vi "Save Direct Summing.vi"(6 "Direct Sum":dbl[](array[numeric]), 7 "Experimental parameters":dbl[](array[numeric]), 8 "Current File Num":u16, 9 "Best Fit Parameters":dbl[](array[numeric]), 10 "Fitting Results Save Path":string, 11 "Fitting Type":u16(ring)) -> ()   [LabVIEW 2015]
uses:
  <vilib>/Utility/file.llb/Read From Spreadsheet File (DBL).vi
  <vilib>/Utility/file.llb/Write To Spreadsheet File (DBL).vi
panel:
  out "Best Fit Parameters 2":dbl[](array[numeric])
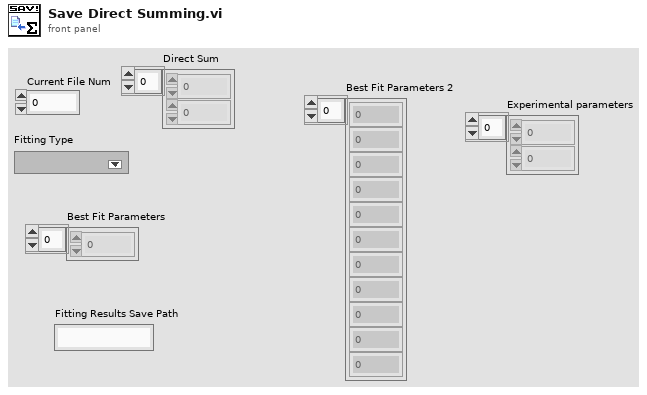
[diagram p1: front panel]
types:
  T1 = enum16{"open", "replace", "create", "open or create", "replace or create", "replace or create with confirmation"}
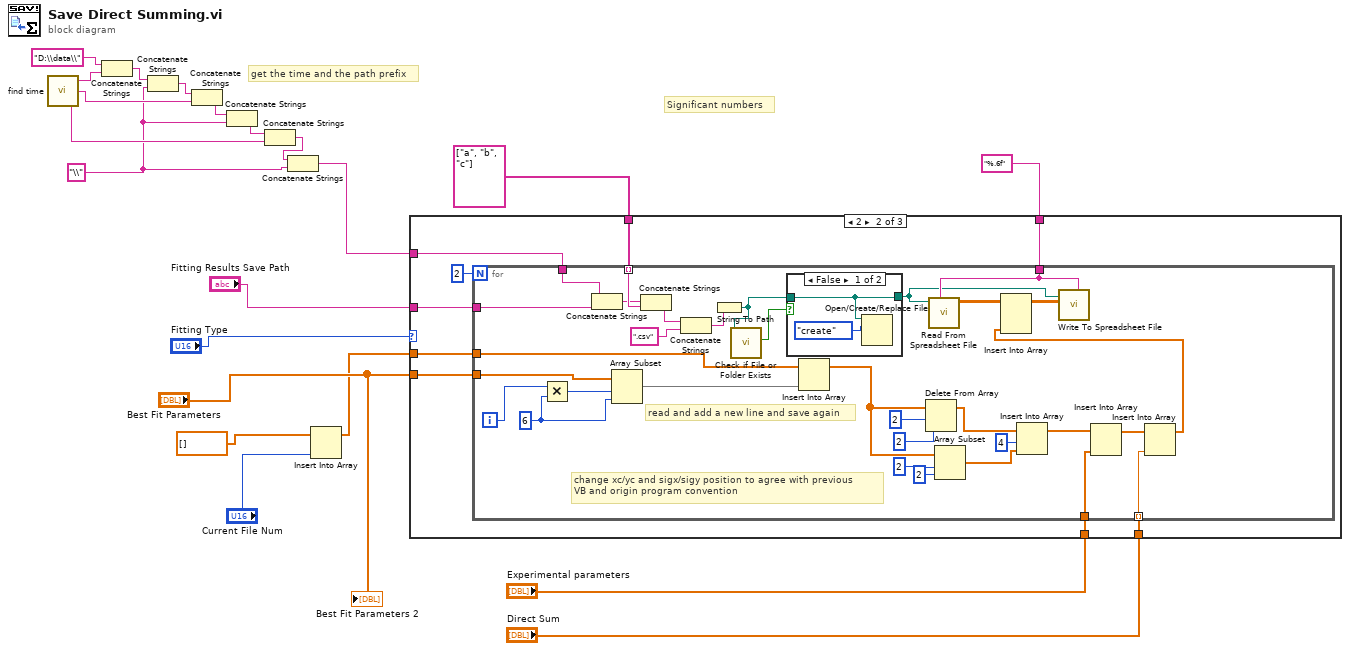
[diagram p0: block diagram]
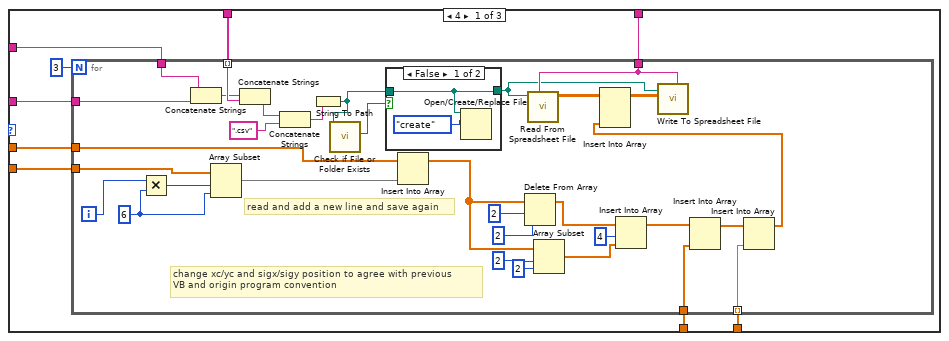
[diagram p2: hidden frame]
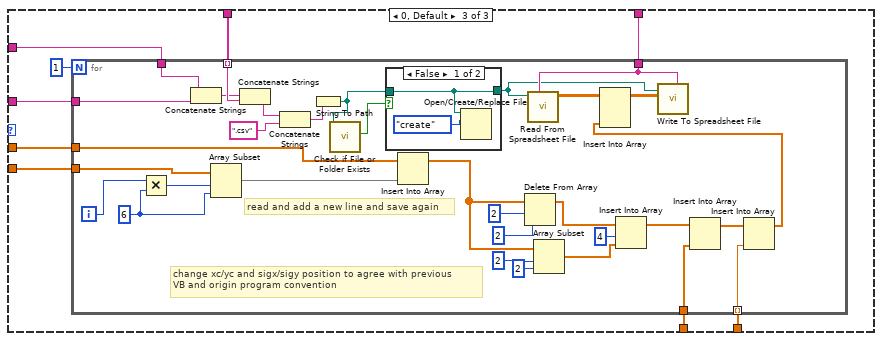
[diagram p5: hidden frame]
diagram:
  w5 = "\\" ("字符串")
  # "get the time and the path prefix"
  # "Significant numbers"
  n1 = call "find time.vi"() -> ("day"=w7:string, "month"=w10:string, "year"=w13:string)  [unwired: 3 in]
  n2 = Concatenate Strings("D:\\data\\", w13) -> (w12:string)
  n3 = Concatenate Strings(w12, w5) -> (w11:string)
  n4 = Concatenate Strings(w11, w10) -> (w9:string)
  n5 = Concatenate Strings(w9, w5) -> (w8:string)
  n6 = Concatenate Strings(w8, w7) -> (w6:string)
  n7 = Concatenate Strings(w6, w5) -> (w4:string)
  n8 = Insert Into Array(array=dbl[] [], new element="Current File Num") -> (w16:dbl[])  [unwired: 1 in]
  n9 = case shown="2" "Fitting Type" {
    tunnel: "Best Fit Parameters" -> [w29 w73 w117]
    tunnel: "Fitting Results Save Path" -> [w28 w72 w116]
    tunnel: w16 -> [w27 w71 w115]
    tunnel: "%.6f" ("format (%.3f)") -> [w26 w70 w114]
    tunnel: w4 -> [w25 w69 w113]
    tunnel: string[] ["a", "b", "c"] ("Fitting Results Save Path") -> [w24 w68 w112]
    tunnel: "Experimental parameters" -> [w23 w67 w111]
    tunnel: "Direct Sum" -> [w22 w66 w110]
    frame 4 {
      n10 = for {
        N: 3 -> [_]
        tunnel: w29 -> [w60]
        tunnel: w28 -> [w31]
        tunnel: w27 -> [w56]
        tunnel: w26 -> [w55]
        tunnel: w25 -> [w54]
        tunnel: w24 -> [w40] mode=indexing
        tunnel: w23 -> [w36]
        tunnel: w22 -> [w34] mode=indexing
        i -> [w32]
        w61 = 6 ("x")
        # "change xc/yc and sigx/sigy position to agree with previous\nVB and origin program convention"
        # "read and add a new line and save again"
        n11 = Multiply(x=w32, y=w61) -> (x*y=w62:i32)
        n12 = Concatenate Strings(w54, w31) -> (w39:string)
        n13 = Array Subset(array=w60, index=w62, length=w61) -> (w57:dbl[])
        n14 = Concatenate Strings(w39, w40) -> (w38:string)
        n15 = Concatenate Strings(w38, ".csv" ("字符串")) -> (w52:string)
        n16 = String To Path(string=w52) -> (path=w50:path)
        n17 = call <vilib>:"Check if File or Folder Exists.vi"("path"=w50) -> ("file or folder exists?"=w51:bool)  [unwired: 8 in, 2 out]
        n18 = case shown="False" w51 {
          tunnel: [w63 w65] -> w49
          tunnel: w50 -> [w63 w65]
          frame False {
            n19 = Open/Create/Replace File(file path (use dialog)=w63, operation (0:open)=T1."create" ("操作(0:open)")) -> ()  [unwired: 4 in, 3 out]
          }
          frame True {
          }
        }
        n20 = Insert Into Array(array=w56, new element=w57) -> (w41:dbl[])  [unwired: 1 in]
        n21 = Delete From Array(array=w41, length=2, index=2) -> (array with subset deleted=w44:dbl[])  [unwired: 1 out]
        n22 = call-poly <vilib>:"Read From Spreadsheet File.vi"("format (%.3f)"=w55, "file path (dialog if empty)"=w49) -> ("all rows"=w59:dbl[][])  [unwired: 5 in, 4 out]
        n23 = Array Subset(array=w41, index=2, length=2) -> (w42:dbl[])
        n24 = Insert Into Array(array=w44, index=4, new element=w42) -> (w37:dbl[])
        n25 = Insert Into Array(array=w37, new element=w36) -> (w35:dbl[])  [unwired: 1 in]
        n26 = Insert Into Array(array=w35, new element=w34) -> (w33:dbl[])  [unwired: 1 in]
        n27 = Insert Into Array(array=w59, new element=w33) -> (w58:dbl[][])  [unwired: 2 in]
        n28 = call-poly <vilib>:"Write To Spreadsheet File.vi"("format (%.3f)"=w55, "2D data"=w58, "file path (dialog if empty)"=w49) -> ()  [unwired: 5 in, 1 out]
      }
    }
    frame 2 {
      n29 = for {
        N: 2 -> [_]
        tunnel: w73 -> [w104]
        tunnel: w72 -> [w75]
        tunnel: w71 -> [w99]
        tunnel: w70 -> [w98]
        tunnel: w69 -> [w97]
        tunnel: w68 -> [w83] mode=indexing
        tunnel: w67 -> [w79]
        tunnel: w66 -> [w77] mode=indexing
        i -> [w103]
        w105 = 6 ("x")
        # "change xc/yc and sigx/sigy position to agree with previous\nVB and origin program convention"
        # "read and add a new line and save again"
        n30 = Multiply(x=w103, y=w105) -> (x*y=w106:i32)
        n31 = Concatenate Strings(w97, w75) -> (w82:string)
        n32 = Array Subset(array=w104, index=w106, length=w105) -> (w100:dbl[])
        n33 = Concatenate Strings(w82, w83) -> (w81:string)
        n34 = Concatenate Strings(w81, ".csv" ("字符串")) -> (w95:string)
        n35 = String To Path(string=w95) -> (path=w93:path)
        n36 = call <vilib>:"Check if File or Folder Exists.vi"("path"=w93) -> ("file or folder exists?"=w94:bool)  [unwired: 8 in, 2 out]
        n37 = case shown="False" w94 {
          tunnel: [w107 w109] -> w92
          tunnel: w93 -> [w107 w109]
          frame False {
            n38 = Open/Create/Replace File(file path (use dialog)=w107, operation (0:open)=T1."create" ("操作(0:open)")) -> ()  [unwired: 4 in, 3 out]
          }
          frame True {
          }
        }
        n39 = Insert Into Array(array=w99, new element=w100) -> (w84:dbl[])  [unwired: 1 in]
        n40 = Delete From Array(array=w84, length=2, index=2) -> (array with subset deleted=w87:dbl[])  [unwired: 1 out]
        n41 = call-poly <vilib>:"Read From Spreadsheet File.vi"("format (%.3f)"=w98, "file path (dialog if empty)"=w92) -> ("all rows"=w102:dbl[][])  [unwired: 5 in, 4 out]
        n42 = Array Subset(array=w84, index=2, length=2) -> (w85:dbl[])
        n43 = Insert Into Array(array=w87, index=4, new element=w85) -> (w80:dbl[])
        n44 = Insert Into Array(array=w80, new element=w79) -> (w78:dbl[])  [unwired: 1 in]
        n45 = Insert Into Array(array=w78, new element=w77) -> (w76:dbl[])  [unwired: 1 in]
        n46 = Insert Into Array(array=w102, new element=w76) -> (w101:dbl[][])  [unwired: 2 in]
        n47 = call-poly <vilib>:"Write To Spreadsheet File.vi"("format (%.3f)"=w98, "2D data"=w101, "file path (dialog if empty)"=w92) -> ()  [unwired: 5 in, 1 out]
      }
    }
    frame 0, Default {
      n48 = for {
        N: 1 -> [_]
        tunnel: w117 -> [w148]
        tunnel: w116 -> [w119]
        tunnel: w115 -> [w143]
        tunnel: w114 -> [w142]
        tunnel: w113 -> [w141]
        tunnel: w112 -> [w127] mode=indexing
        tunnel: w111 -> [w123]
        tunnel: w110 -> [w121] mode=indexing
        i -> [w147]
        w149 = 6 ("x")
        # "change xc/yc and sigx/sigy position to agree with previous\nVB and origin program convention"
        # "read and add a new line and save again"
        n49 = Multiply(x=w147, y=w149) -> (x*y=w150:i32)
        n50 = Concatenate Strings(w141, w119) -> (w126:string)
        n51 = Array Subset(array=w148, index=w150, length=w149) -> (w144:dbl[])
        n52 = Concatenate Strings(w126, w127) -> (w125:string)
        n53 = Concatenate Strings(w125, ".csv" ("字符串")) -> (w139:string)
        n54 = String To Path(string=w139) -> (path=w137:path)
        n55 = call <vilib>:"Check if File or Folder Exists.vi"("path"=w137) -> ("file or folder exists?"=w138:bool)  [unwired: 8 in, 2 out]
        n56 = case shown="False" w138 {
          tunnel: [w151 w153] -> w136
          tunnel: w137 -> [w151 w153]
          frame False {
            n57 = Open/Create/Replace File(file path (use dialog)=w151, operation (0:open)=T1."create" ("操作(0:open)")) -> ()  [unwired: 4 in, 3 out]
          }
          frame True {
          }
        }
        n58 = Insert Into Array(array=w143, new element=w144) -> (w128:dbl[])  [unwired: 1 in]
        n59 = Delete From Array(array=w128, length=2, index=2) -> (array with subset deleted=w131:dbl[])  [unwired: 1 out]
        n60 = call-poly <vilib>:"Read From Spreadsheet File.vi"("format (%.3f)"=w142, "file path (dialog if empty)"=w136) -> ("all rows"=w146:dbl[][])  [unwired: 5 in, 4 out]
        n61 = Array Subset(array=w128, index=2, length=2) -> (w129:dbl[])
        n62 = Insert Into Array(array=w131, index=4, new element=w129) -> (w124:dbl[])
        n63 = Insert Into Array(array=w124, new element=w123) -> (w122:dbl[])  [unwired: 1 in]
        n64 = Insert Into Array(array=w122, new element=w121) -> (w120:dbl[])  [unwired: 1 in]
        n65 = Insert Into Array(array=w146, new element=w120) -> (w145:dbl[][])  [unwired: 2 in]
        n66 = call-poly <vilib>:"Write To Spreadsheet File.vi"("format (%.3f)"=w142, "2D data"=w145, "file path (dialog if empty)"=w136) -> ()  [unwired: 5 in, 1 out]
      }
    }
  }
  "Best Fit Parameters 2" <- "Best Fit Parameters"
